vi "centre_stage.vi"(8 "error in":errorcluster, 10 "handle in":i32, 11 "Destination":dbl) -> (0 "error out":errorcluster, 2 "handle out":i32)   [LabVIEW 2013]
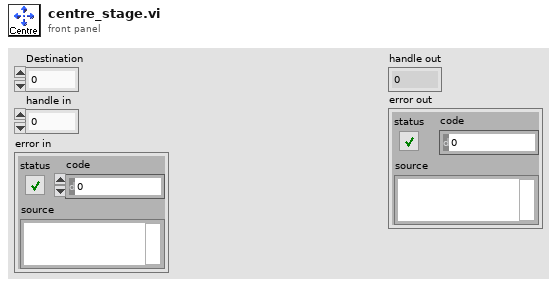
[diagram p1: front panel]
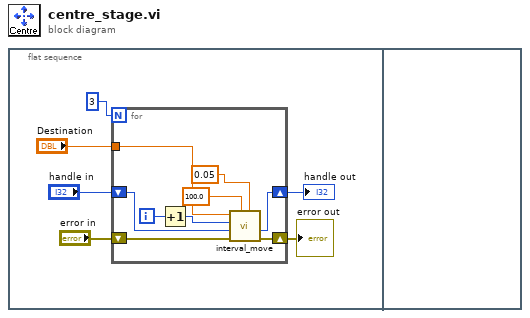
[diagram p0: block diagram]
diagram:
  n1 = flat-sequence {
    frame #0 {
      n2 = for {
        N: 3 -> [_]
        shift-right: [w9] -> w3
        shift-left: "handle in" -> [w13]
        tunnel: "Destination" -> [w14]
        shift-right: [w10] -> w1
        shift-left: "error in" -> [w11]
        i -> [w15]
        n3 = Increment(x=w15) -> (x+1=w12:i32)
        n4 = call "interval_move.vi"("Interval (s)"=0.05, "Speed(um/s)"=100.0, "error in"=w11, "handle"=w13, "axis"=w12, "Destination"=w14) -> ("error out"=w10:errorcluster, "handle out"=w9:i32)  [unwired: 2 in, 2 out]
      }
      "handle out" <- w3
      "error out" <- w1
    }
    frame #1 {
    }
  }
